vi "Polarizer_calib_find_zero_5.vi"(2 "Tolerance":dbl=0.065, 3 "Find Zero":bool, 6 "Medir pasos\n por vuelta":bool, 7 "Angulo \ndeseado":dbl, 8 "Argumento":string="50", 9 "Número de motor":string="1", 10 "Pasos por \nvuelta":dbl=652.0, 11 "Go to angle":bool) -> ()   [LabVIEW 2013]
uses:
  <vilib>/Analysis/baseanly.llb/Mean (DBL).vi
  <vilib>/Utility/file.llb/Write To Spreadsheet File (DBL).vi
  <vilib>/regexp/Match Regular Expression.xnode
  <vilib>/Analysis/NI_AALBase.lvlib
panel:
  in  "wait until completion? (T)":bool=TRUE
  out "i new":i32
  in  "Boolean 2":bool
  in  "Set speed":bool
  in  "Current Step":bool
  in  "Set Zero":bool
  in  "Shutter off":bool
  in  "Shutter on":bool
  in  "Stop":bool
  in  "Go to step":bool
  in  "Constant speed":bool
  in  "Comando":string
  in  "x":bool
  out "x > y?":bool
  in  "Boolean":bool
  out "Array":string[](array[string])
  out "Error":dbl format="%#_4g"
  out "Min value":dbl
  in  "Tab Control":enum32{"Live Picture", "ICImagingControl "}(tab)
  out "Live Picture":picture
  in  "ICImagingControl 2":refnum<k7>(container)
  out "nearest integer value":dbl
  out "Angulo \nrecorrido":dbl
  out "Angulo por\npaso":dbl
  out "Terminal output":string
  in  "Directorio scripts ArduinoStepper.py":path=path "C:/Users/franjas/Documents/rutinas-calibracion-slm"
  out "Comando que está siendo enviado a python":string
  in  "Zero_bol":bool
  out "Current Value":dbl format="%0.2f"
  in  "Save history data":bool
  out "Waveform Chart":dbl(graph)
  out "Found minimum":bool=TRUE
  out "i old":i32
  out "Waveform Chart 2":dbl(graph)
  in  "Stop VI":bool
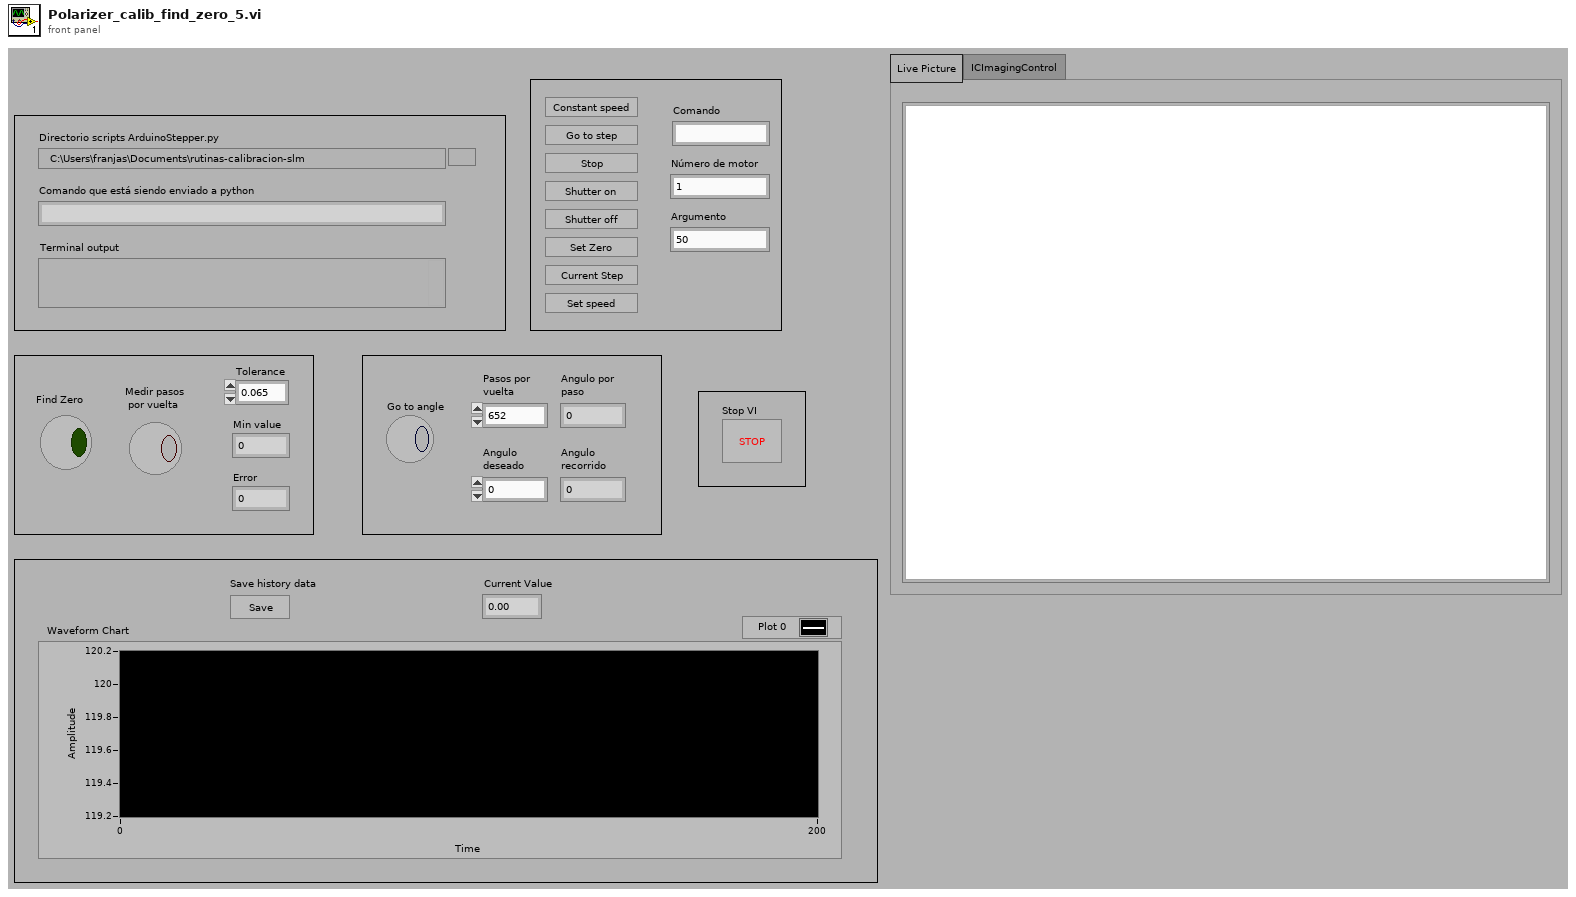
[diagram p1: front panel]
types:
  T1 = typedef "imagedata.ctl" = cluster{"image type":i32, "image depth":i32, "image":u8[], "mask":u8[], "colors":u32[], "Rectangle":cluster{"left":i16, "top":i16, "right":i16, "bottom":i16}}
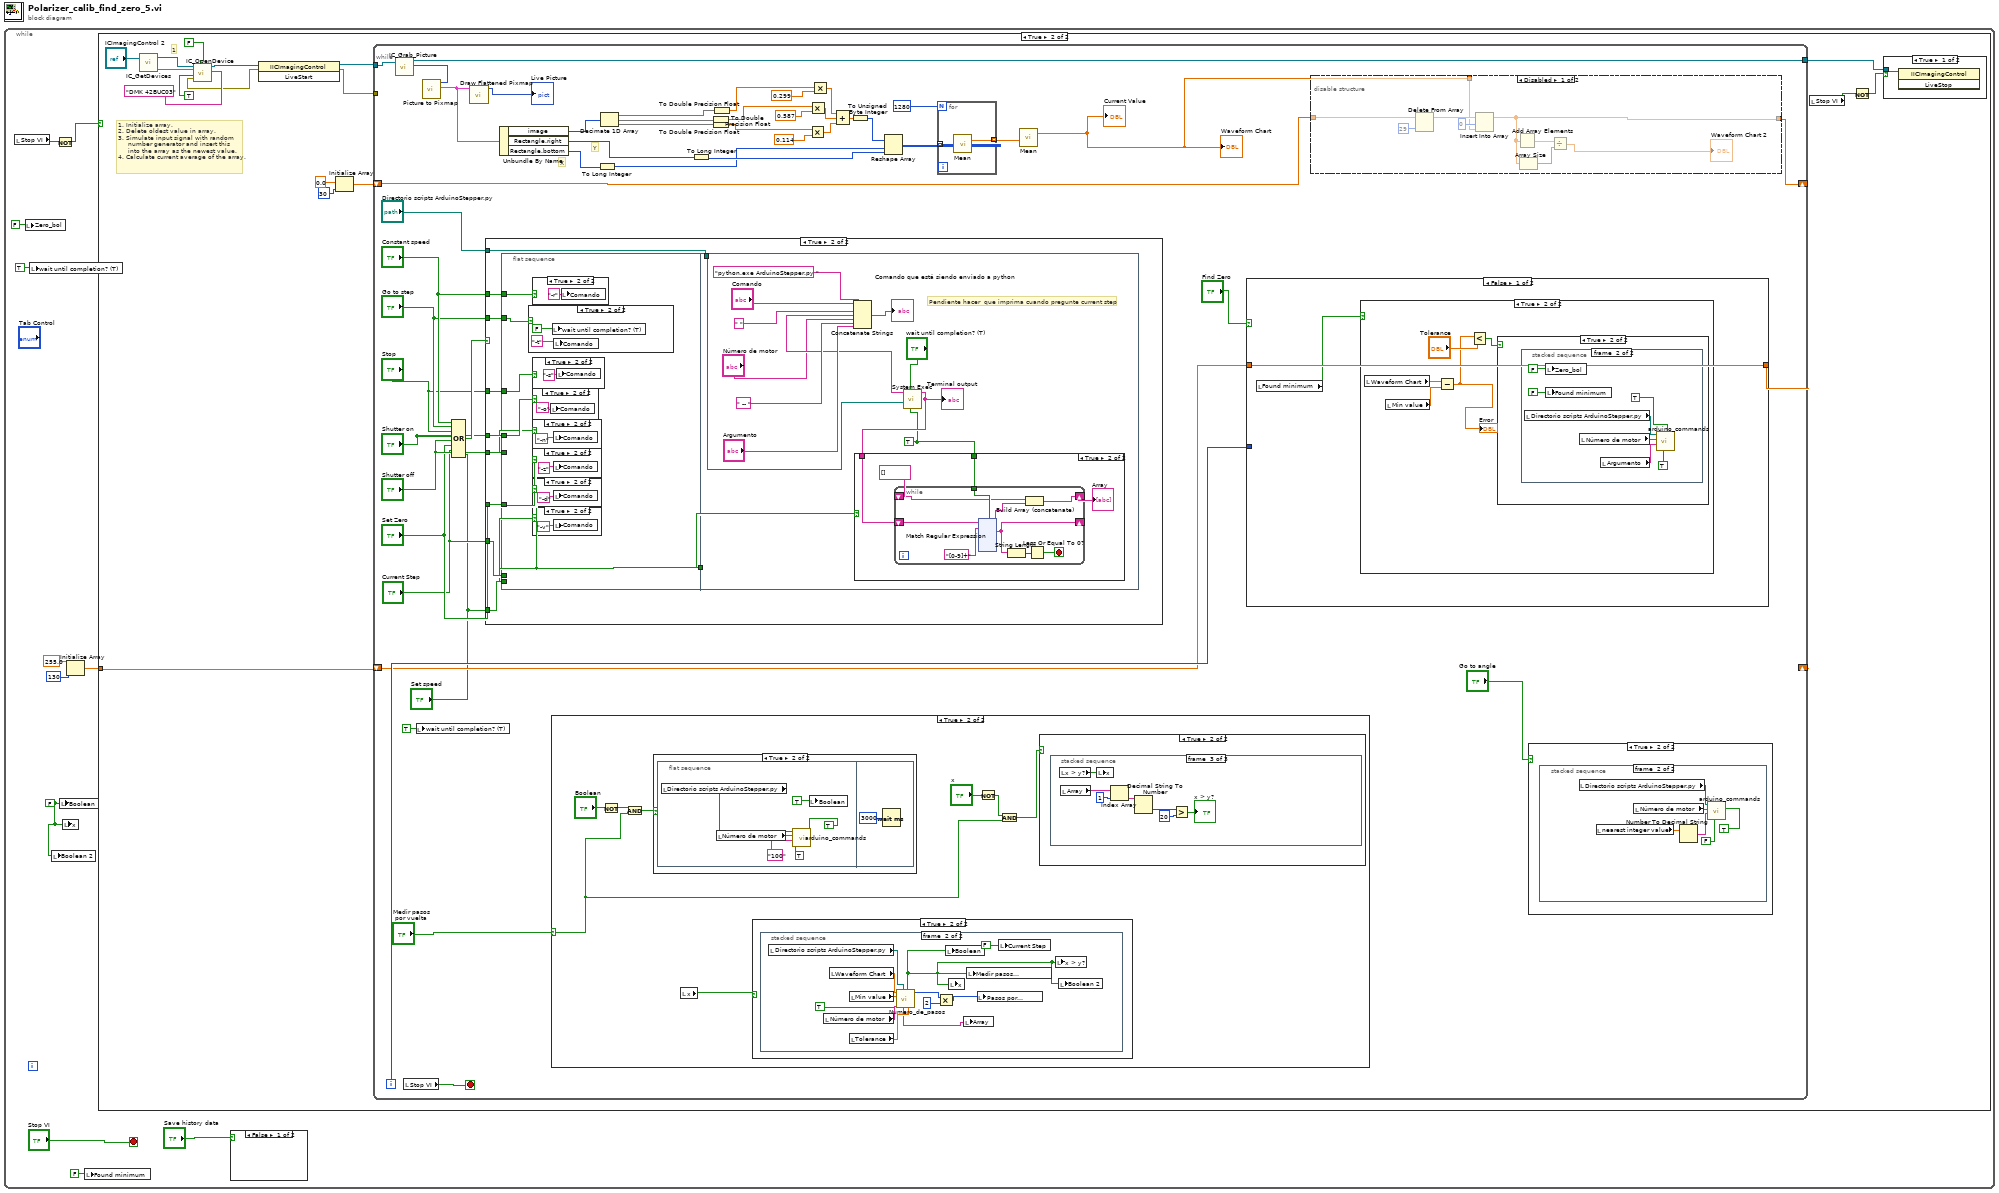
[diagram p0: block diagram]
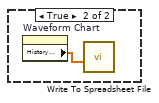
[diagram p2: hidden frame]
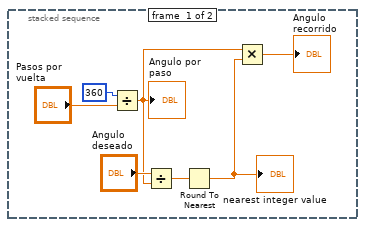
[diagram p5: hidden frame]
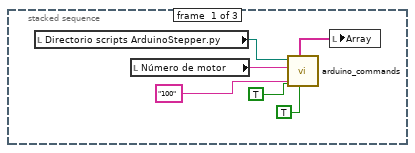
[diagram p8: hidden frame]
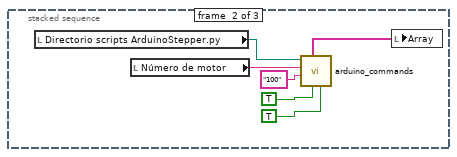
[diagram p9: hidden frame]
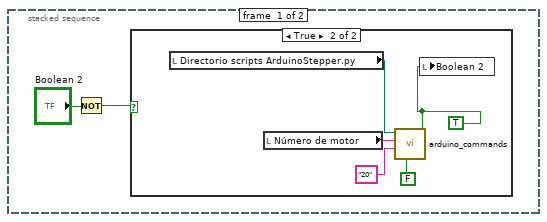
[diagram p12: hidden frame]
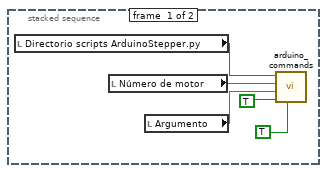
[diagram p17: hidden frame]
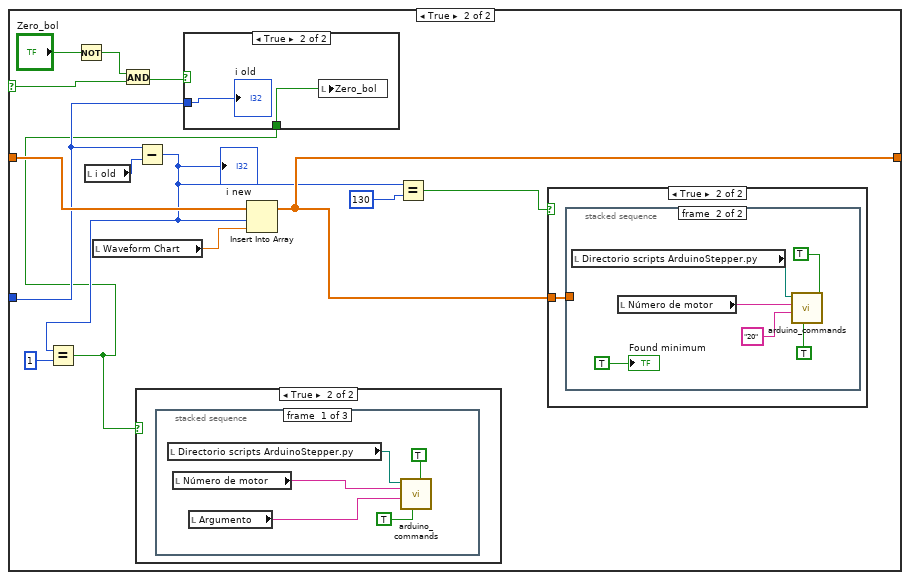
[diagram p18: hidden frame]
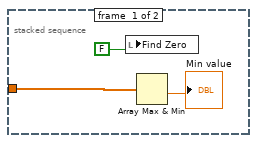
[diagram p20: hidden frame]
diagram:
  n1 = while {
    stop <- "Stop VI" stop-if-true
    w1 = FALSE ("Boolean")
    n2 = local read "Stop VI"() -> (w4:bool)
    n3 = local write "Zero_bol"(FALSE ("Zero_bol")) -> ()
    n4 = local write "wait until completion? (T)"(TRUE ("wait until completion? (T)")) -> ()
    n5 = local write "Boolean 2"(w1) -> ()
    n6 = Not(x=w4) -> (.not. x?=w5:bool)
    n7 = local write "Boolean"(w1) -> ()
    n8 = local write "x"(w1) -> ()
    n9 = Initialize Array(255.0 ("element"), 130 ("dimension size")) -> (w8:dbl[])
    n10 = local write "Found minimum"(FALSE ("Found minimum")) -> ()
    n11 = case shown="True" w5 {
      tunnel: w8 -> [_ w17]
      frame False {
      }
      frame True {
        # "1. Initialize array.\n2. Delete oldest value in array.\n3. Simulate input signal with random\n     number generator and insert this\n     into the array as the newest value.\n4. Calculate current average of the array."
        # "1"
        n12 = call <userlib>:"IC_GetDevices.vi"("ICImagingControl In"="ICImagingControl 2") -> ("ICImagingControl Out"=w27:refnum<k7>, "Error Out"=w23:errorcluster)  [unwired: 1 in, 1 out]
        n13 = call <userlib>:"IC_OpenDevice.vi"("Color"=FALSE, "Error In (no error)"=w23, "Live"=TRUE, "Device"="DMK 42BUC03", "ICImagingControl In"=w27) -> ("ICImagingControl Out"=w24:refnum<k7>, "Error Out"=w22:errorcluster)  [unwired: 1 in, 4 out]
        n14 = invoke class="IICImagingControl" method="LiveStart"(reference=w24, error in=w22) -> (reference out=w16:refnum<k7>, error out=w21:errorcluster)  [unwired: 1 in, 1 out]
        n15 = Initialize Array "Initialize Array"(0.0 ("element"), 30 ("dimension size")) -> (w15:dbl[])
        n16 = while {
          tunnel: w16 -> [w72]
          tunnel: w21 -> [_]
          tunnel: [w73] -> w20
          shift-right: [w49] -> _
          shift-left: w15 -> [w48]
          shift-right: [w46] -> _
          shift-left: w17 -> [w45]
          i -> [w47]
          stop <- w31 stop-if-true
          # "Y"
          # "X"
          n17 = call <userlib>:"IC_Grab_Picture.vi"("ICImagingControl In"=w72) -> ("ICImagingControl Out"=w73:refnum<k7>, "Picture Out"=w77:picture)  [unwired: 1 in, 2 out]
          n18 = local read "Stop VI"() -> (w31:bool)
          n19 = local write "wait until completion? (T)"(TRUE ("wait until completion? (T)")) -> ()
          n20 = call <vilib>:"Picture to Pixmap.vi"("picture"=w77) -> ("image data"=w65:T1)  [unwired: 9 in, 1 out]
          n21 = Compound Arithmetic op=OR("Constant speed", "Go to step", "Stop", "Shutter on", "Shutter off", "Set Zero", "Current Step", "Set speed") -> (w74:bool)
          n22 = call <vilib>:"Draw Flattened Pixmap.vi"("image data"=w65) -> ("new picture"=→"Live Picture":picture)  [unwired: 8 in]
          n23 = case shown="True" w74 {
            tunnel: "Directorio scripts ArduinoStepper.py" -> [_ w223]
            tunnel: "Set Zero" -> [_ w222]
            tunnel: "Constant speed" -> [_ w221]
            tunnel: "Go to step" -> [_ w220]
            tunnel: "Stop" -> [_ w219]
            tunnel: "Shutter on" -> [_ w218]
            tunnel: "Shutter off" -> [_ w217]
            tunnel: "Current Step" -> [_ w216]
            tunnel: "Set speed" -> [_ w214]
            frame False {
            }
            frame True {
              n24 = flat-sequence {
                tunnel: w222 -> [w231]
                tunnel: w221 -> [w230]
                tunnel: w220 -> [w229]
                tunnel: w219 -> [w228]
                tunnel: w218 -> [w227]
                tunnel: w217 -> [w226]
                tunnel: w216 -> [w225]
                tunnel: [w225] -> w215
                tunnel: w214 -> [w224]
                tunnel: w223 -> [w252]
                tunnel: w215 -> [w242]
                frame #0 {
                  n25 = case shown="True" w229 {
                    frame False {
                    }
                    frame True {
                      n26 = local write "wait until completion? (T)"(FALSE ("wait until completion? (T)")) -> ()
                      n27 = local write "Comando"("-t" ("Comando")) -> ()
                    }
                  }
                  n28 = case shown="True" w230 {
                    frame False {
                    }
                    frame True {
                      n29 = local write "Comando"("-r" ("Comando")) -> ()
                    }
                  }
                  n30 = case shown="True" w228 {
                    frame False {
                    }
                    frame True {
                      n31 = local write "Comando"("-s" ("Comando")) -> ()
                    }
                  }
                  n32 = case shown="True" w227 {
                    frame False {
                    }
                    frame True {
                      n33 = local write "Comando"("-o" ("Comando")) -> ()
                    }
                  }
                  n34 = case shown="True" w226 {
                    frame False {
                    }
                    frame True {
                      n35 = local write "Comando"("-n" ("Comando")) -> ()
                    }
                  }
                  n36 = case shown="True" w231 {
                    frame False {
                    }
                    frame True {
                      n37 = local write "Comando"("-z" ("Comando")) -> ()
                    }
                  }
                  n38 = case shown="True" w225 {
                    frame False {
                    }
                    frame True {
                      n39 = local write "Comando"("-d" ("Comando")) -> ()
                    }
                  }
                  n40 = case shown="True" w224 {
                    frame False {
                    }
                    frame True {
                      n41 = local write "Comando"("-v" ("Comando")) -> ()
                    }
                  }
                }
                frame #1 {
                  w243 = TRUE ("run minimized? (F)")
                  # "Pendiente hacer  que imprima cuando pregunte current step"
                  n42 = Concatenate Strings("python.exe ArduinoStepper.py ", "Comando", " " ("string"), "Número de motor", " -- ", "Argumento") -> (w248:string)
                  "Comando que está siendo enviado a python" <- w248
                  n43 = call <vilib>:"System Exec.vi"("run minimized? (F)"=w243, "wait until completion? (T)"="wait until completion? (T)", "working directory"=w252, "command line"=w248) -> ("standard output"=w244:string)  [unwired: 4 in, 3 out]
                  "Terminal output" <- w244
                  n44 = case shown="True" w242 {
                    tunnel: w244 -> [_ w256]
                    tunnel: w243 -> [_ w255]
                    frame False {
                    }
                    frame True {
                      n45 = while {
                        shift-right: [w263] -> _
                        shift-left: w256 -> [w264]
                        tunnel: w255 -> [w260]
                        shift-right: [w259] -> w254
                        shift-left: string[] [] -> [w257]
                        stop <- w261 stop-if-true
                        n46 = xnode "Match Regular Expression"("input string"=w264, "regular expression"="[0-9]+", "multiline? (F)"=w260) -> ("whole match"=w258:string, "after match"=w263:string)  [unwired: 3 in, 5 out]
                        n47 = String Length(string=w263) -> (length=w262:i32)
                        n48 = Build Array (concatenate)(w257, w258) -> (w259:string[])
                        n49 = Less Or Equal To 0?(x=w262) -> (x <= 0?=w261:bool)
                      }
                      "Array" <- w254
                    }
                  }
                }
              }
            }
          }
          n50 = Unbundle By Name(w65) -> ("image"=w53:u8[], "Rectangle.right"=w69:i16, "Rectangle.bottom"=w67:i16)
          n51 = case shown="True" "Medir pasos\n por vuelta" {
            selector: "Medir pasos\n por vuelta" -> [_ w94]
            frame False {
            }
            frame True {
              n52 = Not(x="Boolean") -> (.not. x?=w98:bool)
              n53 = And(x=w98, y=w94) -> (x .and. y?=w96:bool)
              n54 = case shown="True" w96 {
                frame False {
                }
                frame True {
                  n55 = flat-sequence {
                    frame #0 {
                      n56 = local read "Directorio scripts ArduinoStepper.py"() -> (w122:path)
                      n57 = local read "Número de motor"() -> (w121:string)
                      n58 = call "arduino_commands.vi"("Constant speed"=TRUE, "wait until completion? (T)"=TRUE, "Argumento"="100", "Número de motor"=w121, "Directorio scripts ArduinoStepper.py"=w122) -> ()  [unwired: 6 in, 1 out]
                      n59 = local write "Boolean"(TRUE ("Boolean")) -> ()
                    }
                    frame #1 {
                      n60 = Wait (ms)(milliseconds to wait=u32 3000) -> ()  [unwired: 1 out]
                    }
                  }
                }
              }
              n61 = local read "x"() -> (w91:bool)
              n62 = case shown="True" w91 {
                frame False {
                }
                frame True {
                  n63 = stacked-sequence {
                    frame #0 {
                      n64 = Not(x="Boolean 2") -> (.not. x?=w125:bool)
                      n65 = case shown="True" w125 {
                        frame False {
                        }
                        frame True {
                          w128 = TRUE ("Constant speed")
                          n66 = local read "Directorio scripts ArduinoStepper.py"() -> (w130:path)
                          n67 = local read "Número de motor"() -> (w131:string)
                          n68 = call "arduino_commands.vi"("Constant speed"=w128, "wait until completion? (T)"=FALSE, "Argumento"="20", "Número de motor"=w131, "Directorio scripts ArduinoStepper.py"=w130) -> ()  [unwired: 6 in, 1 out]
                          n69 = local write "Boolean 2"(w128) -> ()
                        }
                      }
                    }
                    frame #1 {
                      n70 = local read "Directorio scripts ArduinoStepper.py"() -> (w141:path)
                      n71 = local read "Número de motor"() -> (w140:string)
                      n72 = local read "Waveform Chart"() -> (w143:dbl)
                      n73 = local read "Min value"() -> (w142:dbl)
                      n74 = local read "Tolerance"() -> (w139:dbl)
                      n75 = call "Numero_de_pasos.vi"("Tolerance"=w139, "Directorio scripts ArduinoStepper.py"=w141, "Número de motor"=w140, "Medir pasos por\nvuelta"=TRUE ("Medir pasos por\nvuelta"), "Minimo"=w142, "Valor actual"=w143) -> ("Half rotation"=w136:i32, "Boolean 2"=w133:bool, "Array"=w132:string[])  [unwired: 3 in]
                      n76 = Multiply(x=w136, y=2) -> (x*y=w134:i32)
                      n77 = local write "Boolean"(w133) -> ()
                      n78 = local write "x"(w133) -> ()
                      n79 = local write "Array"(w132) -> ()
                      n80 = local write "Medir pasos\n por vuelta"(w133) -> ()
                      n81 = local write "Pasos por \nvuelta"(w134) -> ()
                      n82 = local write "Current Step"(FALSE ("Current Step")) -> ()
                      n83 = local write "x > y?"(w133) -> ()
                      n84 = local write "Boolean 2"(w133) -> ()
                    }
                  }
                }
              }
              n85 = Not(x="x") -> (.not. x?=w92:bool)
              n86 = And(x=w92, y=w94) -> (x .and. y?=w95:bool)
              n87 = case shown="True" w95 {
                frame False {
                }
                frame True {
                  n88 = stacked-sequence {
                    frame #0 {
                      n89 = local read "Directorio scripts ArduinoStepper.py"() -> (w103:path)
                      n90 = local read "Número de motor"() -> (w104:string)
                      n91 = call "arduino_commands.vi"("wait until completion? (T)"=TRUE, "Stop"=TRUE ("Constant speed"), "Argumento"="100", "Número de motor"=w104, "Directorio scripts ArduinoStepper.py"=w103) -> ("Array"=w102:string[])  [unwired: 6 in]
                      n92 = local write "Array"(w102) -> ()
                    }
                    frame #1 {
                      n93 = local read "Directorio scripts ArduinoStepper.py"() -> (w108:path)
                      n94 = local read "Número de motor"() -> (w109:string)
                      n95 = call "arduino_commands.vi"("Current Step"=TRUE, "wait until completion? (T)"=TRUE, "Argumento"="100", "Número de motor"=w109, "Directorio scripts ArduinoStepper.py"=w108) -> ("Array"=w105:string[])  [unwired: 6 in]
                      n96 = local write "Array"(w105) -> ()
                    }
                    frame #2 {
                      n97 = local read "x > y?"() -> (w113:bool)
                      n98 = local read "Array"() -> (w115:string[])
                      n99 = local write "x"(w113) -> ()
                      n100 = Index Array(array=w115, index=1) -> (element=w114:string)
                      n101 = Decimal String To Number(string=w114) -> (number=w116:i32)  [unwired: 2 in, 1 out]
                      n102 = Greater?(x=w116, y=20) -> (0:→"x > y?":bool)
                    }
                  }
                }
              }
            }
          }
          n103 = To Long Integer(number=w67) -> (32bit integer=w66:i32)
          n104 = Decimate 1D Array(w53) -> (w52:u8[], w51:u8[], w50:u8[])
          n105 = To Long Integer(number=w69) -> (32bit integer=w68:i32)
          n106 = To Double Precision Float(number=w51) -> (double precision float=w62:dbl[])
          n107 = To Double Precision Float(number=w50) -> (double precision float=w61:dbl[])
          n108 = To Double Precision Float(number=w52) -> (double precision float=w63:dbl[])
          n109 = Multiply(x=w61, y=0.114) -> (x*y=w55:dbl[])
          n110 = Multiply(x=w62, y=0.587) -> (x*y=w56:dbl[])
          n111 = Multiply(x=w63, y=0.299) -> (x*y=w57:dbl[])
          n112 = Compound Arithmetic op=ADD(w57, w56, w55) -> (w54:dbl[])
          n113 = To Unsigned Byte Integer(number=w54) -> (unsigned 8bit integer=w70:u8[])
          n114 = Reshape Array(w70, w66, w68) -> (w64:u8[][])
          n115 = for {
            N: 1280 -> [_]
            tunnel: [w384] -> w76 mode=indexing
            tunnel: w64 -> [w383] mode=indexing
            n116 = call-poly <vilib>:"Mean.vi"("X"=w383) -> ("mean"=w384:dbl)  [unwired: 1 out]
          }
          n117 = call-poly <vilib>:"Mean.vi"("X"=w76) -> ("mean"=w37:dbl)  [unwired: 1 out]
          "Waveform Chart" <- w37
          "Current Value" <- w37
          n118 = case shown="False" "Find Zero" {
            selector: "Find Zero" -> [_ w175]
            tunnel: w45 -> [w154 w185]
            tunnel: w47 -> [_ w182]
            tunnel: [w154 w178] -> w46
            frame False {
              n119 = local read "Found minimum"() -> (w153:bool)
              n120 = case shown="True" w153 {
                frame False {
                }
                frame True {
                  n121 = local read "Waveform Chart"() -> (w157:dbl)
                  n122 = local read "Min value"() -> (w159:dbl)
                  n123 = Subtract(x=w157, y=w159) -> (x-y=w155:dbl)
                  "Error" <- w155
                  n124 = Less?(x=w155, y="Tolerance") -> (x < y?=w158:bool)
                  n125 = case shown="True" w158 {
                    frame False {
                    }
                    frame True {
                      n126 = stacked-sequence {
                        frame #0 {
                          n127 = local read "Directorio scripts ArduinoStepper.py"() -> (w164:path)
                          n128 = local read "Número de motor"() -> (w163:string)
                          n129 = local read "Argumento"() -> (w162:string)
                          n130 = call "arduino_commands.vi"("wait until completion? (T)"=TRUE, "Stop"=TRUE, "Argumento"=w162, "Número de motor"=w163, "Directorio scripts ArduinoStepper.py"=w164) -> ()  [unwired: 6 in, 1 out]
                        }
                        frame #1 {
                          n131 = local read "Directorio scripts ArduinoStepper.py"() -> (w171:path)
                          n132 = local write "Zero_bol"(FALSE ("zero_bol")) -> ()
                          n133 = local write "Found minimum"(FALSE ("Found minimum")) -> ()
                          n134 = local read "Número de motor"() -> (w170:string)
                          n135 = local read "Argumento"() -> (w169:string)
                          n136 = call "arduino_commands.vi"("Set zero"=TRUE, "wait until completion? (T)"=TRUE, "Argumento"=w169, "Número de motor"=w170, "Directorio scripts ArduinoStepper.py"=w171) -> ()  [unwired: 6 in, 1 out]
                        }
                      }
                    }
                  }
                }
              }
            }
            frame True {
              n137 = Not(x="Zero_bol") -> (.not. x?=w177:bool)
              n138 = local read "i old"() -> (w174:i32)
              n139 = local read "Waveform Chart"() -> (w184:dbl)
              n140 = And(x=w177, y=w175) -> (x .and. y?=w183:bool)
              n141 = Subtract(x=w182, y=w174) -> (x-y=w173:i32)
              "i new" <- w173
              n142 = Equal?(x=w173, y=1) -> (x = y?=w172:bool)
              n143 = case shown="True" w172 {
                frame False {
                }
                frame True {
                  n144 = stacked-sequence {
                    frame #0 {
                      n145 = local read "Directorio scripts ArduinoStepper.py"() -> (w200:path)
                      n146 = local read "Número de motor"() -> (w199:string)
                      n147 = local read "Argumento"() -> (w198:string)
                      n148 = call "arduino_commands.vi"("Set zero"=TRUE, "wait until completion? (T)"=TRUE, "Argumento"=w198, "Número de motor"=w199, "Directorio scripts ArduinoStepper.py"=w200) -> ()  [unwired: 6 in, 1 out]
                    }
                    frame #1 {
                      n149 = local read "Directorio scripts ArduinoStepper.py"() -> (w205:path)
                      n150 = local read "Número de motor"() -> (w204:string)
                      n151 = call "arduino_commands.vi"("Constant speed"=TRUE ("Set zero"), "wait until completion? (T)"=FALSE, "Argumento"="50", "Número de motor"=w204, "Directorio scripts ArduinoStepper.py"=w205) -> ()  [unwired: 6 in, 1 out]
                    }
                    frame #2 {
                      n152 = local read "Directorio scripts ArduinoStepper.py"() -> (w211:path)
                      n153 = local read "Número de motor"() -> (w210:string)
                      n154 = Number To Decimal String(number=-400 ("dimension size")) -> (decimal integer string=w207:string)  [unwired: 1 in]
                      n155 = call "arduino_commands.vi"("Go to step"=TRUE, "wait until completion? (T)"=FALSE, "Argumento"=w207, "Número de motor"=w210, "Directorio scripts ArduinoStepper.py"=w211) -> ()  [unwired: 6 in, 1 out]
                    }
                  }
                }
              }
              n156 = case shown="True" w183 {
                tunnel: w182 -> [_ w213]
                tunnel: w172 -> [_ w212]
                frame False {
                }
                frame True {
                  n157 = local write "Zero_bol"(w212) -> ()
                  "i old" <- w213
                }
              }
              n158 = Insert Into Array(array=w185, index=w173, new element=w184) -> (w178:dbl[])
              n159 = Equal?(x=w173, y=130) -> (x = y?=w180:bool)
              n160 = case shown="True" w180 {
                tunnel: w178 -> [_ w186]
                frame False {
                }
                frame True {
                  n161 = stacked-sequence {
                    tunnel: w186 -> [w188 _]
                    frame #0 {
                      n162 = local write "Find Zero"(FALSE ("Zero")) -> ()
                      n163 = Array Max & Min(array=w188) -> (min value=→"Min value":dbl)  [unwired: 3 out]
                    }
                    frame #1 {
                      n164 = local read "Directorio scripts ArduinoStepper.py"() -> (w195:path)
                      n165 = local read "Número de motor"() -> (w194:string)
                      n166 = call "arduino_commands.vi"("Constant speed"=TRUE, "wait until completion? (T)"=TRUE, "Argumento"="20", "Número de motor"=w194, "Directorio scripts ArduinoStepper.py"=w195) -> ()  [unwired: 6 in, 1 out]
                      "Found minimum" <- TRUE ("Found minimum")
                    }
                  }
                }
              }
            }
          }
          n167 = disable-structure shown="Disabled" {
            disable-tunnel: [w148 _] -> w49
            disable-tunnel: w48 -> [w147 _]
            disable-tunnel: w37 -> [w146 _]
            frame Disabled {
              n168 = Delete From Array "Delete From Array"(array=w147, index=29) -> (array with subset deleted=w152:dbl[])  [unwired: 1 in, 1 out]
              n169 = Insert Into Array "Insert Into Array"(array=w152, index=0, new element=w146) -> (w148:dbl[])
              n170 = Add Array Elements(numeric array=w148) -> (sum=w149:dbl)
              n171 = Array Size(array=w148) -> (size(s)=w145:i32)
              n172 = Divide(x=w149, y=w145) -> (x/y=→"Waveform Chart 2":dbl)
            }
            frame Enabled {
            }
          }
          n173 = case shown="True" "Go to angle" {
            frame False {
            }
            frame True {
              n174 = stacked-sequence {
                frame #0 {
                  n175 = Divide(x=360, y="Pasos por \nvuelta") -> (x/y=w79:dbl)
                  "Angulo por\npaso" <- w79
                  n176 = Divide(x="Angulo \ndeseado", y=w79) -> (x/y=w81:dbl)
                  n177 = Round To Nearest(number=w81) -> (nearest integer value=w80:dbl)
                  "nearest integer value" <- w80
                  n178 = Multiply(x=w79, y=w80) -> (x*y=→"Angulo \nrecorrido":dbl)
                }
                frame #1 {
                  n179 = local read "Directorio scripts ArduinoStepper.py"() -> (w90:path)
                  n180 = local read "nearest integer value"() -> (w86:dbl)
                  n181 = local read "Número de motor"() -> (w89:string)
                  n182 = Number To Decimal String(number=w86) -> (decimal integer string=w87:string)  [unwired: 1 in]
                  n183 = call "arduino_commands.vi"("Go to step"=TRUE, "wait until completion? (T)"=FALSE, "Argumento"=w87, "Número de motor"=w89, "Directorio scripts ArduinoStepper.py"=w90) -> ()  [unwired: 6 in, 1 out]
                }
              }
            }
          }
        }
        n184 = local read "Stop VI"() -> (w14:bool)
        n185 = Not(x=w14) -> (.not. x?=w13:bool)
        n186 = case shown="True" w13 {
          tunnel: w20 -> [w385 _]
          frame True {
            n187 = invoke class="IICImagingControl" method="LiveStop"(reference=w385) -> ()  [unwired: 2 in, 3 out]
          }
          frame False {
          }
        }
      }
    }
    n188 = case shown="False" "Save history data" {
      frame False {
      }
      frame True {
        n189 = property on="Waveform Chart" class="WFChart (strict)"() -> ("History Data"=w12:dbl[])  [unwired: 2 in, 2 out]
        n190 = call-poly <vilib>:"Write To Spreadsheet File.vi"("1D data"=w12) -> ()  [unwired: 7 in, 1 out]
      }
    }
  }
